vi "Error.vi"(2 "error in (no error)":errorcluster, 3 "error in (no error) 2":errorcluster) -> (0 "error out":errorcluster)   [LabVIEW 2014]
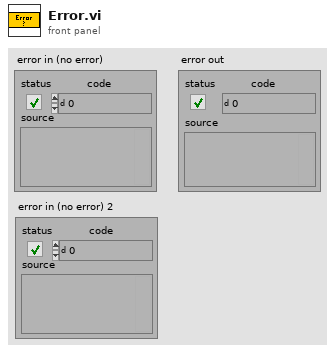
[diagram p1: front panel]
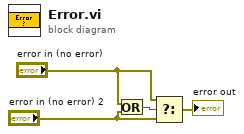
[diagram p0: block diagram]
diagram:
  n1 = Or(x="error in (no error)", y="error in (no error) 2") -> (x .or. y?=w4:bool)
  n2 = Select(t="error in (no error)", s=w4, f="error in (no error) 2") -> (s? t:f=→"error out":errorcluster)
